vi "leds.vi"(0 "LED Robot Mode":T1(ring), 1 "Opening Ceremonies Mode":bool, 2 "Override?":bool, 3 "LEDs Off?":bool) -> ()   [LabVIEW 2014]
uses:
  <vilib>/Rock Robotics/Network Tables/NT Write Boolean.vi
  <vilib>/Rock Robotics/Network Tables/NT Write Number.vi
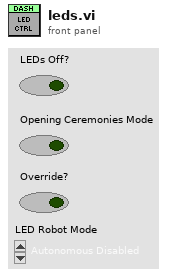
[diagram p1: front panel]
types:
  T1 = enum16{"Autonomous Disabled", "Autonomous Enabled", "Teleop Disabled", "Teleop Enabled", "Disconnected", "Finish", "Test Disabled", "Test Enabled", "Emergency Stopped"}
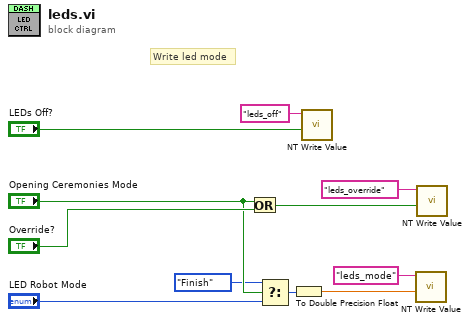
[diagram p0: block diagram]
diagram:
  # "Write led mode"
  n1 = Or(x="Opening Ceremonies Mode", y="Override?") -> (x .or. y?=w6:bool)
  n2 = Select(t=T1."Finish", s="Opening Ceremonies Mode", f="LED Robot Mode") -> (s? t:f=w2:T1)
  n3 = To Double Precision Float(number=w2) -> (double precision float=w1:dbl)
  n4 = call-poly <vilib>:"NT Write Value.vi"("Boolean"="LEDs Off?", "Name"="leds_off") -> ()  [unwired: 9 in, 1 out]
  n5 = call-poly <vilib>:"NT Write Value.vi"("Numeric"=w1, "Name"="leds_mode") -> ()  [unwired: 9 in, 1 out]
  n6 = call-poly <vilib>:"NT Write Value.vi"("Boolean"=w6, "Name"="leds_override") -> ()  [unwired: 9 in, 1 out]
